vi "Format & Precision Dialog.vi"(8 "Error In":errorcluster, 11 "Display Format in":T1) -> (0 "Error Out":errorcluster, 1 "Cancelled?":bool, 3 "Display Format out":T1)   [LabVIEW 2021, in "GUI.lvlib"]
uses:
  GUI.lvlib
  Numeric Display Format.ctl
  <vilib>/Utility/miscctls.llb/LVFormatAndPrecisionTypeDef.ctl
panel:
  in  "Precision":u8
  in  "Numeric Display Format":T2=enum."Scientific"
  in  "Input Message":string
  out "Message":string
  in  "Cancel":bool
  in  "OK":bool
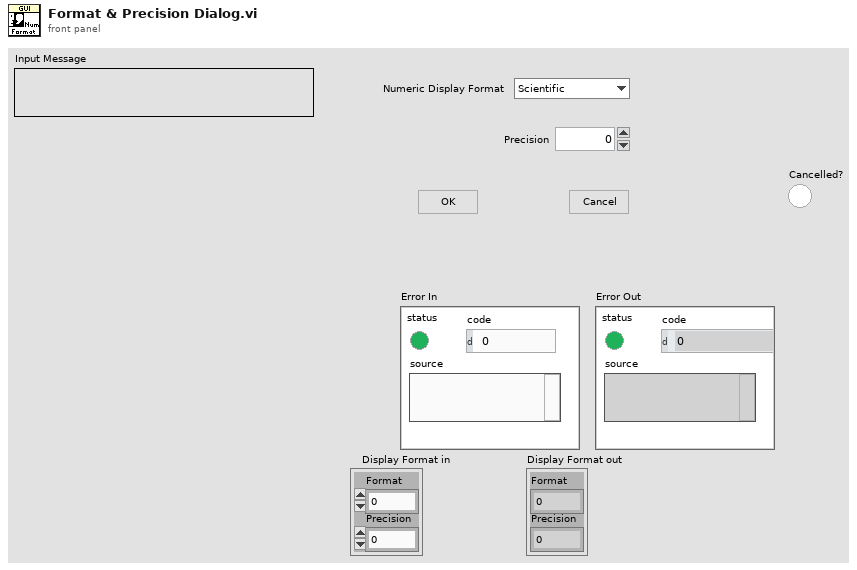
[diagram p1: front panel]
types:
  T1 = typedef "LVFormatAndPrecisionTypeDef.ctl" = cluster{"Format":u8, "Precision":u8}
  T2 = typedef "GUI.lvlib/Numeric Display Format.ctl" = enum16{"Decimal", "Scientific", "Engineering", "Binary", "Octal", "Hexadecimal", "Relative tie", "Time and Date", "SI"}
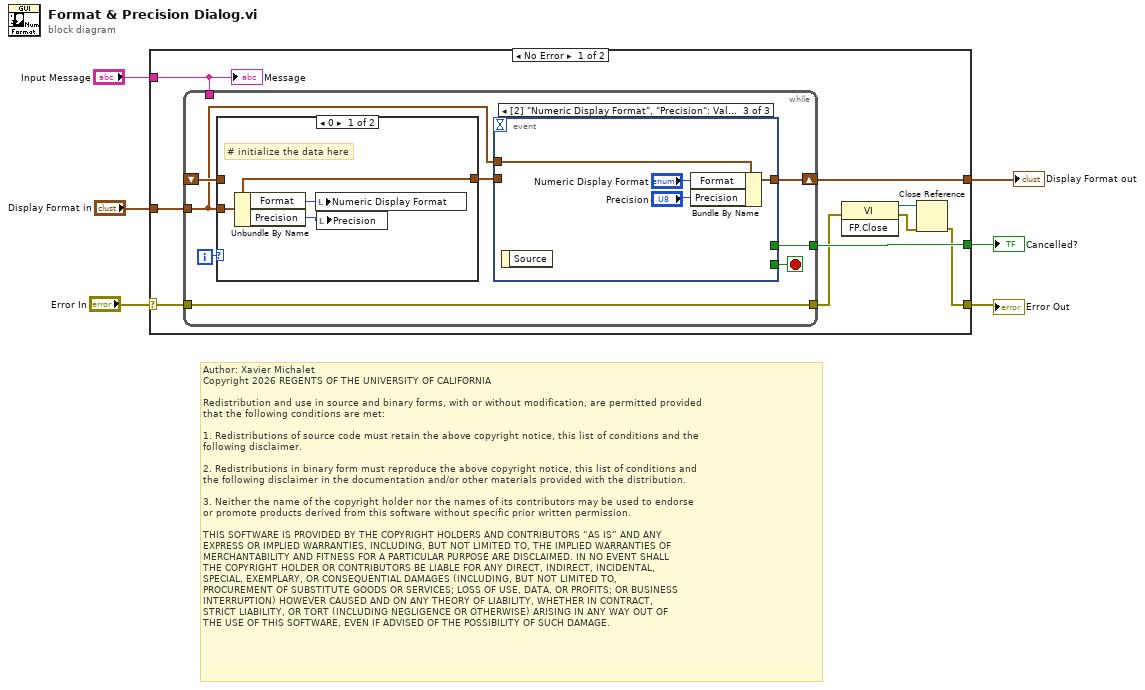
[diagram p0: block diagram]
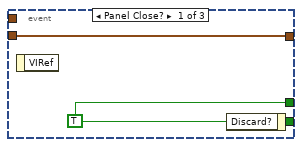
[diagram p3: hidden frame]
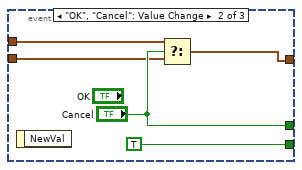
[diagram p4: hidden frame]
diagram:
  # "Author: Xavier Michalet\nCopyright 2026 REGENTS OF THE UNIVERSITY OF CALIFORNIA\n\nRedistribution and use in source and binary forms, with or without modification, are permitted provided\nthat the following conditions are met:\n\n1. Redistributions of source code must retain the above copyright notice, this list of conditions and the\nfollowing disclaimer.\n\n2. Redistributions in binary form must reproduce the above copyright notice, this list of conditions and\nthe following disclaimer in the documentation and/or other materials provided with the distribution.\n\n3. Neither the name of the copyright holder nor the names of its contributors may be used to endorse \nor promote products derived from this software without specific prior written permission.\n\nTHIS SOFTWARE IS PROVIDED BY THE COPYRIGHT HOLDERS AND CONTRIBUTORS “AS IS” AND ANY \nEXPRESS OR IMPLIED WARRANTIES, INCLUDING, BUT NOT LIMITED TO, THE IMPLIED WARRANTIES OF\nMERCHANTABILITY AND FITNESS FOR A PARTICULAR PURPOSE ARE DISCLAIMED. IN NO EVENT SHALL\nTHE COPYRIGHT HOLDER OR CONTRIBUTORS BE LIABLE FOR ANY DIRECT, INDIRECT, INCIDENTAL, \nSPECIAL, EXEMPLARY, OR CONSEQUENTIAL DAMAGES (INCLUDING, BUT NOT LIMITED TO, \nPROCUREMENT OF SUBSTITUTE GOODS OR SERVICES; LOSS OF USE, DATA, OR PROFITS; OR BUSINESS\nINTERRUPTION) HOWEVER CAUSED AND ON ANY THEORY OF LIABILITY, WHETHER IN CONTRACT, \nSTRICT LIABILITY, OR TORT (INCLUDING NEGLIGENCE OR OTHERWISE) ARISING IN ANY WAY OUT OF\nTHE USE OF THIS SOFTWARE, EVEN IF ADVISED OF THE POSSIBILITY OF SUCH DAMAGE."
  n1 = case shown="No Error" "Error In" {
    selector: "Error In" -> [w9 w39]
    tunnel: [w15 _] -> w6
    tunnel: [w14 _] -> w1
    tunnel: "Input Message" -> [w13 _]
    tunnel: [w10 w39] -> w3
    tunnel: "Display Format in" -> [w7 _]
    frame No Error {
      n2 = while {
        tunnel: [w22] -> w15
        shift-right: [w19] -> w14
        shift-left: _ -> [w20]
        tunnel: w13 -> [_]
        tunnel: w9 -> [w17]
        tunnel: [w17] -> w8
        tunnel: w7 -> [w16]
        i -> [w21]
        stop <- w23 stop-if-true
        n3 = case shown="0" w21 {
          tunnel: w20 -> [_ w27]
          tunnel: [w24 w27] -> w18
          tunnel: w16 -> [w24 _]
          frame 0 {
            # "# initialize the data here"
            n4 = Unbundle By Name(w24) -> ("Format"=w25:u8, "Precision"=w26:u8)
            n5 = local write "Numeric Display Format"(w25) -> ()
            n6 = local write "Precision"(w26) -> ()
          }
          frame 1, Default {
          }
        }
        n7 = event shown="[2] \"Numeric Display Format\", \"Precision\": Value Change" {
          selector: _ -> [_ _ _]
          dyn-events: _ -> [_ _ _]
          timeout: _ -> [_ _ _]
          tunnel: [w29 TRUE ("Discard?") _] -> w23
          tunnel: [w29 "Cancel" _] -> w22
          tunnel: [w28 w30 w37] -> w19
          tunnel: w18 -> [w28 w32 _]
          tunnel: w16 -> [_ w31 w38]
          event Panel Close? {
            w29 = TRUE ("Discard?")
            n8 = event-data() -> ()  [unwired: 1 in, 1 out]
            n9 = event-data("Discard?"=w29) -> ()  [unwired: 1 in, 1 out]
          }
          event "OK", "Cancel": Value Change {
            n10 = event-data() -> ()  [unwired: 1 in, 1 out]
            n11 = Select(t=w31, s="Cancel", f=w32) -> (s? t:f=w30:T1)
          }
          event "Precision": Value Change {
            n12 = event-data() -> ()  [unwired: 1 in, 1 out]
            n13 = Bundle By Name(cluster=w38, "Format"="Numeric Display Format", "Precision"="Precision") -> (w37:T1)
          }
        }
      }
      n14 = invoke class="VI" method="FP.Close"(error in=w8) -> (reference out=w12:refnum<vi>, error out=w11:errorcluster)  [unwired: 2 in, 1 out]
      n15 = Close Reference(reference=w12, error in (no error)=w11) -> (error out=w10:errorcluster)
      "Message" <- w13
    }
    frame Error {
    }
  }
  "Cancelled?" <- w6
  "Error Out" <- w3
  "Display Format out" <- w1
